vi "Agilent PNA Read Data3.vi"(0 "VISA session":refnum<visa-resource-name>="GPIB0::16::INSTR", 5 "Format":string(combo)="MLINear", 7 "Measurement Name (MY_MEAS)":string="MY_MEAS", 9 "Sample Count (401)":u32=201, 11 "Error In (no error)":errorcluster) -> (4 "dup VISA session":refnum<visa-resource-name>="GPIB0::16::INSTR", 6 "Data":dbl[](array[numeric])=[-0.00338059138317, 0.00741421633493, -0.05359599108, -0.0741992219194, 0.0277704867168, 0.0683540120135, -0.0573406064067, -0.160668168542, -0.0540431157295, 0.0345875887534, -0.0799611020497, -0.18001950941, -0.00238919194139, 0.0530245757153, -0.0796482390852, -0.21103500402, -0.094310246197, 0.0746020319771, 0.0396637384069, -0.130934166741, -0.0844453321769, 0.0466949680104, -0.0324728144639, -0.188198400335, -0.121677372585, 0.0832686541384, 0.0878249846831, -0.159796032908, -0.265343585685, -0.151147927336, -0.130607844279, -0.243809915923, -0.2519823243, -0.18345319126, -0.294166293281, -0.487756028752, -0.385899362075, -0.142102960372, -0.147951546917, -0.367572173399, -0.381284791948, -0.2100913072, -0.185274064794, -0.326641273647, -0.240418410005, -0.069095891841, -0.116041326911, -0.36073919432, -0.392092890151, -0.281413932165, -0.296065336463, -0.397066504298, -0.278126091552, -0.0606534407394, -0.203082697367, -0.480067035172, -0.268606009438, 0.240587615827, 0.359350113419, 0.0469284592863, 0.172290997484, 0.662211667451, 0.580624295662, -0.0368954309438, -0.0313769044643, 0.773961624934, 1.12194261593, 0.512876778539, 0.0940033845348, 0.272631193578, 0.487315941282, 0.4137606839, 0.56037884426, 0.945092138384, 0.893138304227, 0.171155951149, -0.242939345039, 0.0872911168954, 0.498050494684, 0.384497139785, 0.0452162140175, -0.000603968519945, 0.00531424747513, -0.25196628691, -0.345664273453, 0.029335473324, 0.343874772215, 0.241780774293, 0.193990580884, 0.373546157564, 0.202577167845, -0.162263482656, -0.0318840048699, 0.242654188648, 0.0626144978636, -0.272994602525, -0.255163320808, -0.564966548754, -1.06053009028, -1.13144950519, -0.611043000005, -0.170158547108, -0.295007698988, -0.580285777185, -0.47659660564, -0.169972226693, -0.0973008194236, -0.102777192489, 0.29788876727, 0.755698994193, 0.177868418447, -1.0208440785, -0.833325409841, 0.421096331639, 0.843196266004, -0.450938954722, -1.26019465575, -0.626426216289, 0.0991627059849, -0.0524276348841, -0.266317557623, -0.0542343540215, -0.0749420060446, -0.438160356472, -0.466948969985, -0.0821814149976, 0.284064883966, 0.402728124159, -0.00911544683979, -0.19044071474, -0.141015385374, -0.0438159354306, -0.0595078767465, 0.269092231077, 0.753443752037, 0.55637889818, -0.0914986873143, -0.0901925965955, 0.353357889948, 0.242885383989, -0.0861157023708, 0.100094344829, 0.315705078038, 0.109854155307, -0.120046908221, -0.297716824793, -0.616475821134, -0.552249880824, 0.0957490217823, 0.483387029276, -0.103412146964, -0.896322827864, -0.947950349698, -0.604975726364, -0.532853738705, -0.667719963134, -0.824433234802, -0.538978193257, -0.439385499951, -0.560715625558, -0.628449470819, -0.200750600218, 0.20147191034, -0.101597641647, -0.498166706421, 0.00612033894372, 0.699980014388, 0.219035922271, -0.887083957618, -1.07131978147, -0.623574677825, -0.45339639732, -0.476151919962, -0.427323053358, -0.471082760815, -0.513935639601, -0.419336575416, -0.396260034206, -0.237334576575, 0.554514503443, 1.4203093752, 1.35280206129, 0.655736420712, 0.322216813142, 0.459069034219, 0.753957297715, 1.08867855925, 1.21225055579, 0.877262835091, 0.282647014111, -0.235889563141, -0.425194428229, 0.00156566179441, 0.747480415509, 0.856063570874, 0.234880053589, -0.094031138628, 0.0738614851684, -0.0224000228021, -0.205488158846, 0.391071948557] format="%.4f", 15 "Error Out":errorcluster)   [LabVIEW 2018]
doc: "This VI configures the sweep parameters and reads data from the analyzer.\n\nNote: To see the data on the analyzer after running the program, from the front panel click: Trace - Math/Memory - Memory Trace"
uses:
  Agilent PNA Series/Agilent PNA Series.lvlib
panel:
  out "波形图":dbl[](graph)=[-0.00338059138317, 0.00741421633493, -0.05359599108, -0.0741992219194, 0.0277704867168, 0.0683540120135, -0.0573406064067, -0.160668168542, -0.0540431157295, 0.0345875887534, -0.0799611020497, -0.18001950941, -0.00238919194139, 0.0530245757153, -0.0796482390852, -0.21103500402, -0.094310246197, 0.0746020319771, 0.0396637384069, -0.130934166741, -0.0844453321769, 0.0466949680104, -0.0324728144639, -0.188198400335, -0.121677372585, 0.0832686541384, 0.0878249846831, -0.159796032908, -0.265343585685, -0.151147927336, -0.130607844279, -0.243809915923, -0.2519823243, -0.18345319126, -0.294166293281, -0.487756028752, -0.385899362075, -0.142102960372, -0.147951546917, -0.367572173399, -0.381284791948, -0.2100913072, -0.185274064794, -0.326641273647, -0.240418410005, -0.069095891841, -0.116041326911, -0.36073919432, -0.392092890151, -0.281413932165, -0.296065336463, -0.397066504298, -0.278126091552, -0.0606534407394, -0.203082697367, -0.480067035172, -0.268606009438, 0.240587615827, 0.359350113419, 0.0469284592863, 0.172290997484, 0.662211667451, 0.580624295662, -0.0368954309438, -0.0313769044643, 0.773961624934, 1.12194261593, 0.512876778539, 0.0940033845348, 0.272631193578, 0.487315941282, 0.4137606839, 0.56037884426, 0.945092138384, 0.893138304227, 0.171155951149, -0.242939345039, 0.0872911168954, 0.498050494684, 0.384497139785, 0.0452162140175, -0.000603968519945, 0.00531424747513, -0.25196628691, -0.345664273453, 0.029335473324, 0.343874772215, 0.241780774293, 0.193990580884, 0.373546157564, 0.202577167845, -0.162263482656, -0.0318840048699, 0.242654188648, 0.0626144978636, -0.272994602525, -0.255163320808, -0.564966548754, -1.06053009028, -1.13144950519, -0.611043000005, -0.170158547108, -0.295007698988, -0.580285777185, -0.47659660564, -0.169972226693, -0.0973008194236, -0.102777192489, 0.29788876727, 0.755698994193, 0.177868418447, -1.0208440785, -0.833325409841, 0.421096331639, 0.843196266004, -0.450938954722, -1.26019465575, -0.626426216289, 0.0991627059849, -0.0524276348841, -0.266317557623, -0.0542343540215, -0.0749420060446, -0.438160356472, -0.466948969985, -0.0821814149976, 0.284064883966, 0.402728124159, -0.00911544683979, -0.19044071474, -0.141015385374, -0.0438159354306, -0.0595078767465, 0.269092231077, 0.753443752037, 0.55637889818, -0.0914986873143, -0.0901925965955, 0.353357889948, 0.242885383989, -0.0861157023708, 0.100094344829, 0.315705078038, 0.109854155307, -0.120046908221, -0.297716824793, -0.616475821134, -0.552249880824, 0.0957490217823, 0.483387029276, -0.103412146964, -0.896322827864, -0.947950349698, -0.604975726364, -0.532853738705, -0.667719963134, -0.824433234802, -0.538978193257, -0.439385499951, -0.560715625558, -0.628449470819, -0.200750600218, 0.20147191034, -0.101597641647, -0.498166706421, 0.00612033894372, 0.699980014388, 0.219035922271, -0.887083957618, -1.07131978147, -0.623574677825, -0.45339639732, -0.476151919962, -0.427323053358, -0.471082760815, -0.513935639601, -0.419336575416, -0.396260034206, -0.237334576575, 0.554514503443, 1.4203093752, 1.35280206129, 0.655736420712, 0.322216813142, 0.459069034219, 0.753957297715, 1.08867855925, 1.21225055579, 0.877262835091, 0.282647014111, -0.235889563141, -0.425194428229, 0.00156566179441, 0.747480415509, 0.856063570874, 0.234880053589, -0.094031138628, 0.0738614851684, -0.0224000228021, -0.205488158846, 0.391071948557]
  # "(c) 2005-2015 National Instruments.  ALL RIGHTS RESERVED."
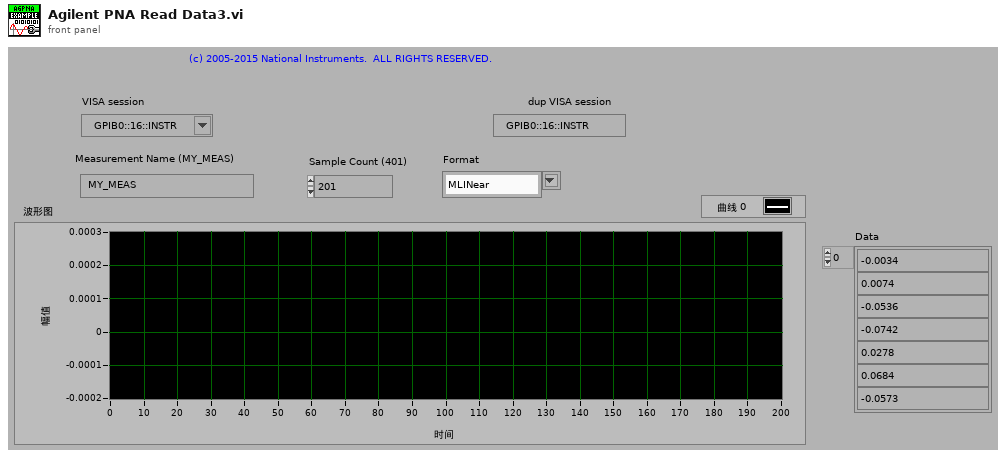
[diagram p1: front panel]
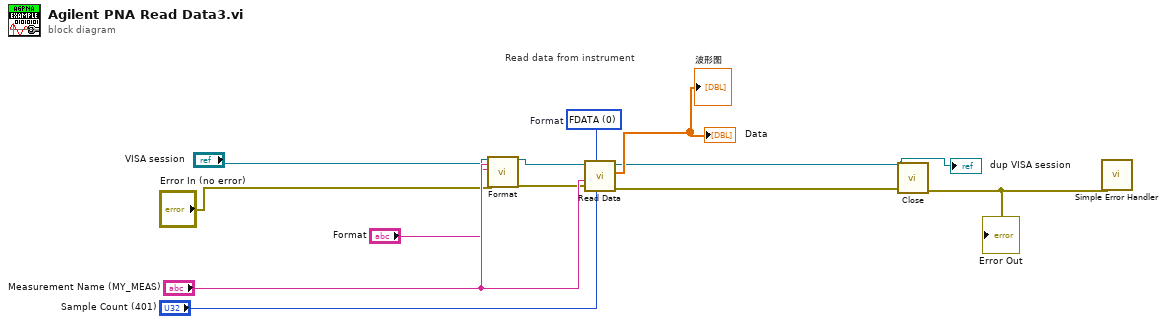
[diagram p0: block diagram]
diagram:
  w12 = u16 0 items=["FDATA", "SDATA", "FMEM", "SMEM", "SDIV"]  # Format
  # "Read data from instrument"
  n1 = call "Format.vi"("VISA IN"="VISA session", "Measurement Name"="Measurement Name (MY_MEAS)", "Format"="Format", "error in"="Error In (no error)") -> ("VISA Out"=w4:refnum<visa-resource-name>, "error out"=w3:errorcluster)  [unwired: 14 in]
  n2 = call "Read Data.vi"("Sample Count (401)"="Sample Count (401)", "Format  (0: FDATA)"=w12, "Error In (no error)"=w3, "Measurement Name (MY_MEAS)"="Measurement Name (MY_MEAS)", "VISA Resource Name"=w4) -> ("Error Out"=w11:errorcluster, "Data"=→"Data" →"波形图":dbl[], "VISA Resource Name Out"=w8:refnum<visa-resource-name>)  [unwired: 4 in]
  "dup VISA session" <- w8
  n3 = call "Close.vi"("Error In (no error)"=w11, "VISA Resource Name"=w8) -> ("Error Out"=w10:errorcluster)  [unwired: 9 in]
  "Error Out" <- w10
  n4 = call <vilib>:"Simple Error Handler.vi"("error in (no error)"=w10) -> ()  [unwired: 4 in, 5 out]
